vi "convert 1D image array to 2D image - double input.vi"(8 "Height":i64(slide)=1200 min=0 max=1200 step=4 scale=0.0..1200.0, 9 "Width":i64(slide)=1920 min=0 max=1920 step=4 scale=0.0..1920.0, 11 "Image Data Array":dbl[](array[numeric])) -> (3 "Intensity Graph":dbl[][](graph))   [LabVIEW 2019]
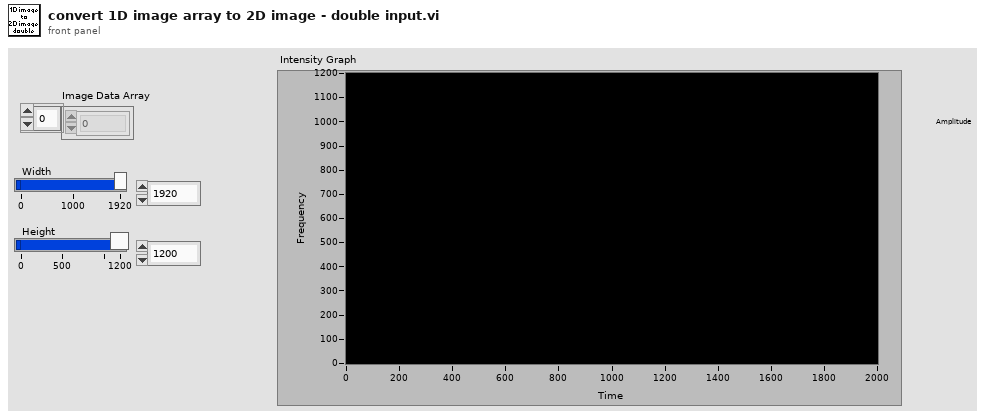
[diagram p1: front panel]
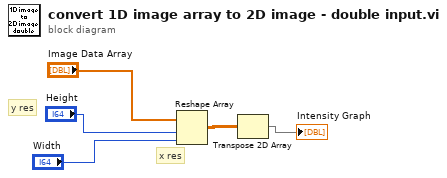
[diagram p0: block diagram]
diagram:
  # "x res"
  # "y res"
  n1 = Reshape Array("Image Data Array", "Height", "Width") -> (w5:dbl[][])
  n2 = Transpose 2D Array(2D array=w5) -> (transposed array=→"Intensity Graph":dbl[][])
